vi "BMark_PositionRadioButtons.vi"(8 "error in (no error)":errorcluster, 11 "RadioButtonsControl in":refnum<vi>) -> (0 "error out":errorcluster)   [LabVIEW 2016]
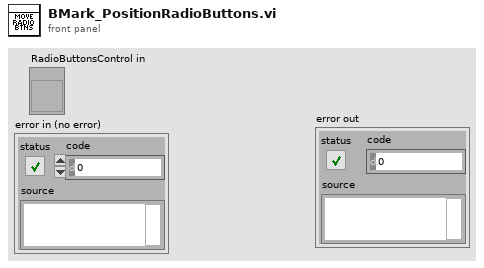
[diagram p1: front panel]
types:
  T1 = typedef "LVPointTypeDef.ctl" = cluster{"Horizontal":i16, "Vertical":i16}
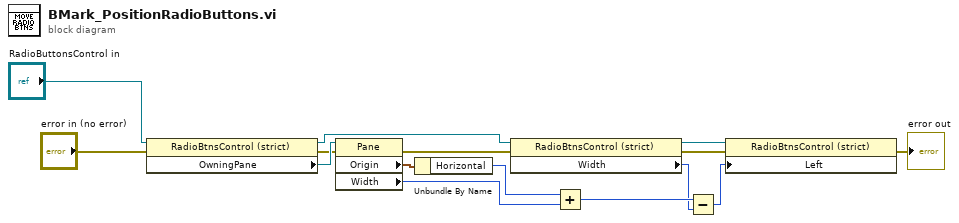
[diagram p0: block diagram]
diagram:
  n1 = property class="RadioBtnsControl (strict)"(reference="RadioButtonsControl in", error in="error in (no error)") -> (reference out=w14:refnum<vi>, error out=w3:errorcluster, "OwningPane"=w13:refnum<vi>)
  n2 = property class="Pane"(reference=w13, error in=w3) -> (error out=w2:errorcluster, "Origin"=w12:T1, "Width"=w10:u32)  [unwired: 1 out]
  n3 = Unbundle By Name(w12) -> ("Horizontal"=w11:i16)
  n4 = property class="RadioBtnsControl (strict)"(reference=w14, error in=w2) -> (reference out=w7:refnum<vi>, error out=w1:errorcluster, "Width"=w8:u32)
  n5 = Add(x=w11, y=w10) -> (x+y=w9:u32)
  n6 = Subtract(x=w9, y=w8) -> (x-y=w6:u32)
  n7 = property class="RadioBtnsControl (strict)"(reference=w7, error in=w1, "Left"=w6) -> (error out=→"error out":errorcluster)  [unwired: 1 out]
